vi "Construct GenericSerializable Instance.vi"(7 "InstanceID":string, 10 "Boolean Data":bool, 11 "Numeric Data":dbl) -> (3 "GenericSerializable out":refnum<class "GenericSerializable.lvclass">)   [LabVIEW 2017, in "Logger Examples.lvlib" / "GenericSerializable.lvclass"]
uses:
  <vilib>/gpm_packages/@cs/event-logger/Examples/GenericSerializable/GenericSerializable.lvclass
  <vilib>/gpm_packages/@cs/event-logger/Examples/GenericSerializable/GenericSerializable.lvclass/GenericSerializable.ctl
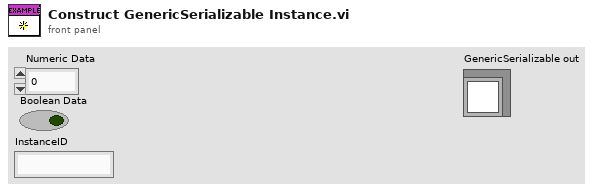
[diagram p1: front panel]
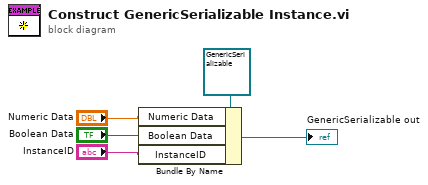
[diagram p0: block diagram]
diagram:
  n1 = Bundle By Name(cluster=refnum<class "GenericSerializable.lvclass"> refnum ("GenericSerializable in"), "Numeric Data"="Numeric Data", "Boolean Data"="Boolean Data", "InstanceID"="InstanceID") -> (→"GenericSerializable out":refnum<class "GenericSerializable.lvclass">)
